vi "Acquisition_Engine.vi"(2 "Tared Input":T1, 3 "queue out 2":refnum<queue>, 4 "Input":T1, 5 "Log Cluster":T2, 6 "notifier out":refnum<notifier>, 7 "DAQmx Error":errorcluster, 8 "queue":refnum<queue>, 9 "Card Samples Per Loop":i32=100 caption="Numeric", 10 "task out":refnum<k21>) -> ()   [LabVIEW 2018]
uses:
  Notifier_control.ctl
  cluster_enum.ctl
  <vilib>/DAQmx/read.llb/DAQmx Read (Analog 1D Wfm NChan NSamp).vi
  <vilib>/DAQmx/miscellaneous.llb/DAQmx Fill In Error Info.vi
  <resource>/objmgr/daqmx.rc
panel:
  out "Card":waveform(dbl)[](graph) caption="Waveform Chart"
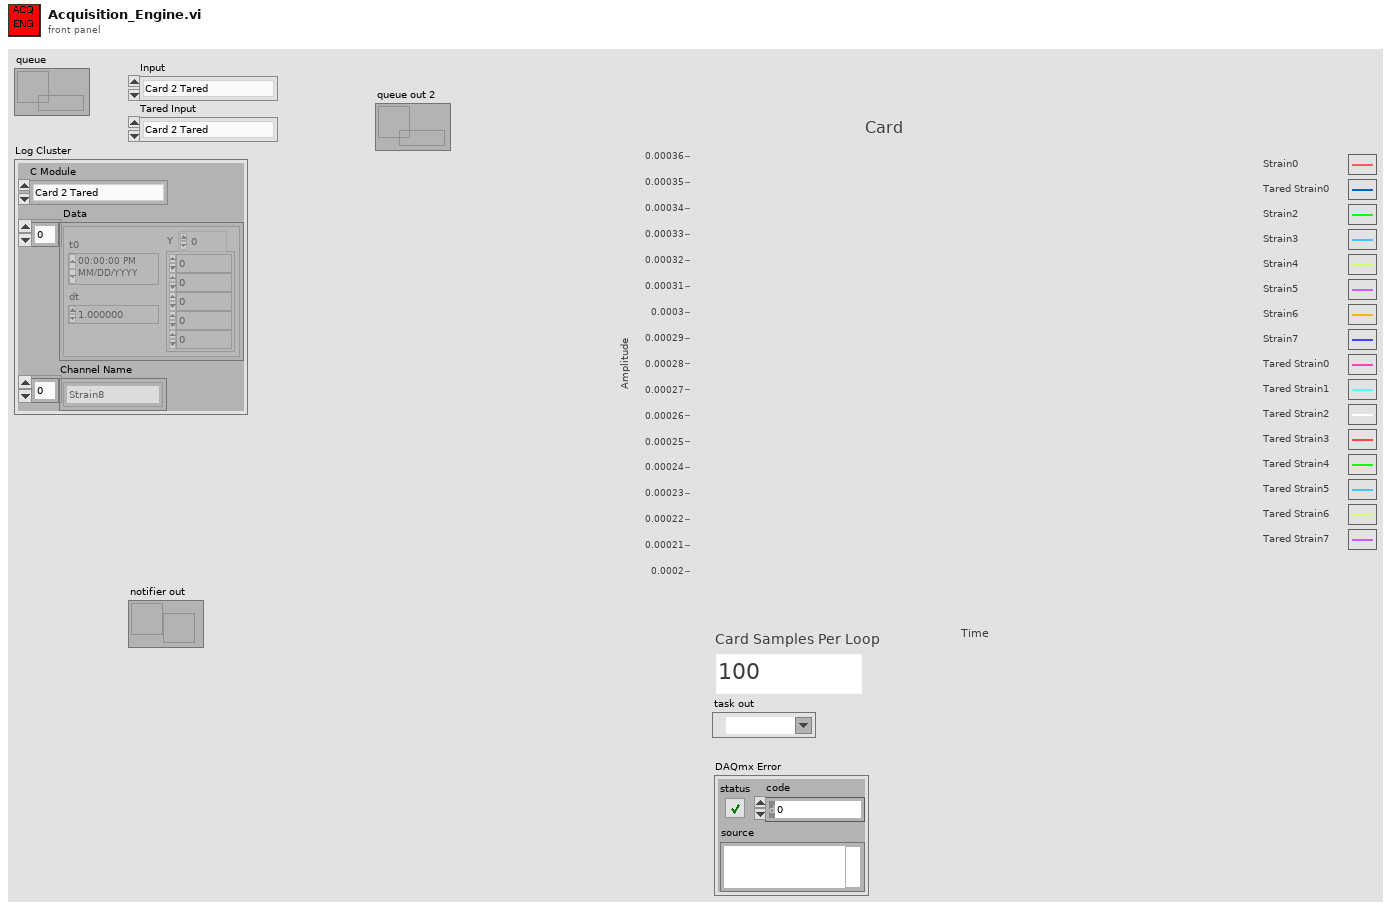
[diagram p1: front panel]
types:
  T1 = typedef "cluster_enum.ctl" = enum16{"Card 2 Tared", "Card 2", "Card 1 Tared", "Card 1"}
  T2 = cluster{"C Module":T1, " Data":waveform(dbl)[], "Channel Name":string[]}
  T3 = typedef "Notifier_control.ctl" = enum16{"Quit", "Run", "Tare", "Save"}
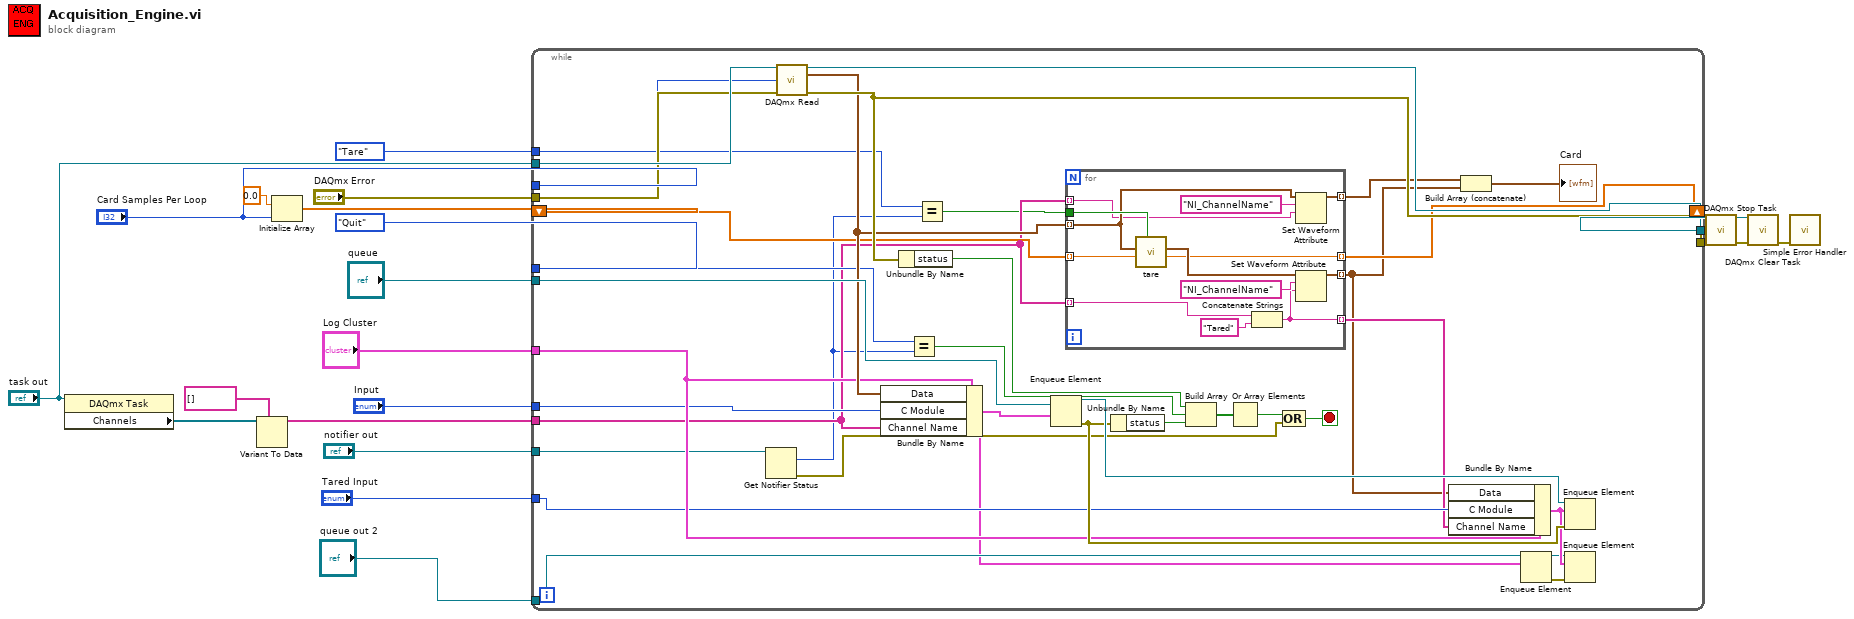
[diagram p0: block diagram]
diagram:
  n1 = property class="DAQmx Task"(reference="task out") -> ("Channels"=w7:refnum<k21>[])  [unwired: 1 in, 2 out]
  n2 = Variant To Data(type=string[] [], Variant=w7) -> (data=w5:string[])  [unwired: 1 in, 1 out]
  n3 = Initialize Array(0.0 ("element"), "Card Samples Per Loop") -> (w16:dbl[])
  n4 = while {
    tunnel: "task out" -> [w54]
    tunnel: [w57] -> w19
    tunnel: "DAQmx Error" -> [w53]
    tunnel: [w51] -> w18
    tunnel: "queue" -> [w50]
    tunnel: "Log Cluster" -> [w42]
    tunnel: "Card Samples Per Loop" -> [w45]
    shift-right: [w43] -> _
    shift-left: w16 -> [w44]
    tunnel: "notifier out" -> [w41]
    tunnel: Notifier_control."Quit" -> [w40]
    tunnel: "Input" -> [w35]
    tunnel: "Tared Input" -> [w34]
    tunnel: w5 -> [w32]
    tunnel: "queue out 2" -> [w28]
    tunnel: Notifier_control."Tare" -> [w24]
    stop <- w36 stop-if-true
    n5 = Get Notifier Status(notifier=w41) -> (current notification=w23:T3, error out=w37:errorcluster)  [unwired: 1 in, 3 out]
    n6 = call-poly <vilib>:"DAQmx Read.vi"("task/channels in"=w54, "number of samples per channel"=w45, "error in"=w53) -> ("task out"=w57:refnum<k21>, "data"=w47:waveform(dbl)[], "error out"=w51:errorcluster)  [unwired: 10 in]
    n7 = Bundle By Name(cluster=w42, "Data"=w47, "C Module"=w35, "Channel Name"=w32) -> (w26:T2)
    n8 = Unbundle By Name(w51) -> ("status"=w56:bool)
    n9 = Equal?(x=w40, y=w23) -> (x = y?=w39:bool)
    n10 = Equal?(x=w24, y=w23) -> (x = y?=w22:bool)
    n11 = Enqueue Element(queue=w50, element=w26) -> (queue out=w49:refnum<queue>, error out=w48:errorcluster)  [unwired: 2 in, 1 out]
    n12 = for {
      tunnel: w47 -> [w68] mode=indexing
      tunnel: [w64] -> w31 mode=indexing
      tunnel: w22 -> [w70]
      tunnel: w32 -> [w58] mode=indexing
      tunnel: [w67] -> w46 mode=indexing
      tunnel: w44 -> [w63] mode=indexing
      tunnel: [w62] -> w43 mode=indexing
      tunnel: w32 -> [w60] mode=indexing
      tunnel: [w59] -> w33 mode=indexing
      n13 = call "tare.vi"("Tare Control"=w70, "Shift Registor"=w63, "Input Waveform"=w68) -> ("Shift Registor Out"=w62:dbl, "output waveform"=w66:waveform(dbl))  [unwired: 7 in]
      n14 = Concatenate Strings(w60, "Tared" ("string")) -> (w59:string)
      n15 = Set Waveform Attribute(5:w58, 6:"NI_ChannelName" ("name"), 7:w68) -> (3:w67:waveform(dbl))  [unwired: 1 in, 2 out]
      n16 = Set Waveform Attribute(5:w59, 6:"NI_ChannelName" ("name"), 7:w66) -> (3:w64:waveform(dbl))  [unwired: 1 in, 2 out]
    }
    n17 = Unbundle By Name(w48) -> ("status"=w52:bool)
    n18 = Build Array(w56, w39, w52) -> (w55:bool[])
    n19 = Or Array Elements(Boolean array=w55) -> (logical OR=w38:bool)
    n20 = Compound Arithmetic op=OR(w38, w37) -> (w36:bool)
    n21 = Bundle By Name(cluster=w42, "Data"=w31, "C Module"=w34, "Channel Name"=w33) -> (w29:T2)
    n22 = Build Array (concatenate)(w46, w31) -> (→"Card":waveform(dbl)[])
    n23 = Enqueue Element(queue=w28, element=w26) -> (queue out=w25:refnum<queue>, error out=w27:errorcluster)  [unwired: 2 in, 1 out]
    n24 = Enqueue Element(queue=w49, element=w29, error in (no error)=w48) -> ()  [unwired: 1 in, 3 out]
    n25 = Enqueue Element(queue=w25, element=w29, error in (no error)=w27) -> ()  [unwired: 1 in, 3 out]
  }
  n26 = call <vilib>:"DAQmx Stop Task.vi"("task/channels in"=w19, "error in"=w18) -> ("task out"=w21:refnum<k21>, "error out"=w20:errorcluster)  [unwired: 12 in]
  n27 = call <vilib>:"DAQmx Clear Task.vi"("task in"=w21, "error in"=w20) -> ("error out"=w17:errorcluster)  [unwired: 13 in]
  n28 = call <vilib>:"Simple Error Handler.vi"("error in (no error)"=w17) -> ()  [unwired: 1 in, 8 out]
